vi "读取生成xhtml.vi"(8 "error in (no error)":errorcluster caption="错误输入（无错误）", 11 "EPUB输入":refnum<class "EPUB.lvclass">) -> (0 "error out":errorcluster caption="错误输出", 2 "xhtml":string[](array[string]), 3 "EPUB输出":refnum<class "EPUB.lvclass">)   [LabVIEW 2016, in "EPUB.lvclass"]
uses:
  EPUB.lvclass
  EPUB.lvclass/EPUB.ctl
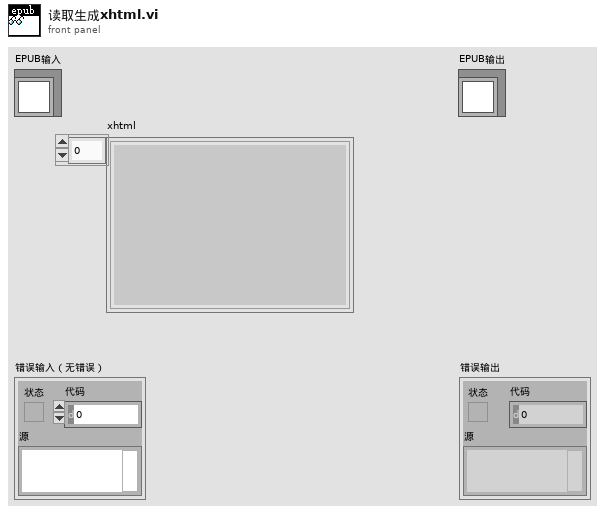
[diagram p1: front panel]
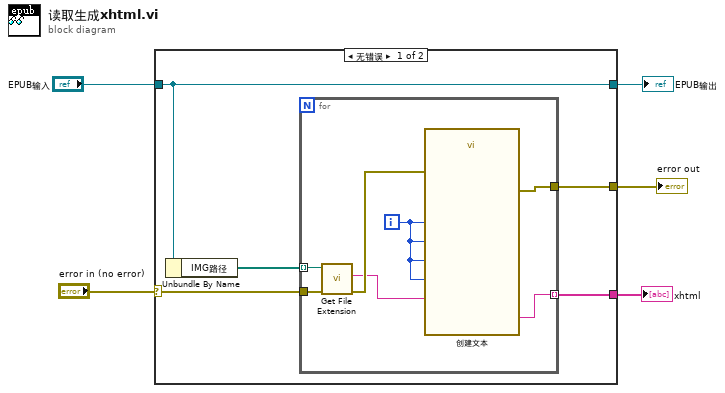
[diagram p0: block diagram]
diagram:
  n1 = case shown="无错误" "error in (no error)" {
    selector: "error in (no error)" -> [w9 w18]
    tunnel: [w8 w18] -> w4
    tunnel: [w10 w19] -> w2
    tunnel: "EPUB输入" -> [w10 w19]
    tunnel: [w7 _] -> w1
    frame No Error {
      n2 = Unbundle By Name(w10) -> ("IMG路径"=w6:path[])
      n3 = for {
        tunnel: w6 -> [w13] mode=indexing
        tunnel: w9 -> [w16]
        tunnel: [w15] -> w8
        tunnel: [w14] -> w7 mode=indexing
        i -> [w12]
        n4 = call <vilib>:"Get File Extension.vi"("error in (no error)"=w16, "file"=w13) -> ("error out"=w17:errorcluster, "lowercase file extension"=w11:string)  [unwired: 5 in, 3 out]
        n5 = call "创建文本"("extname"=w11, "idx3"=w12, "idx"=w12, "idx1"=w12, "error in (no error)"=w17, "idx2"=w12) -> ("Result"=w14:string, "error out"=w15:errorcluster)  [unwired: 8 in]
      }
    }
    frame Error {
    }
  }
  "error out" <- w4
  "EPUB输出" <- w2
  "xhtml" <- w1
